vi "ReadMicaCSV.vi"() -> ()   [LabVIEW 2018]
uses:
  <vilib>/ErrorRing/Error Ring.xnode
panel:
  in  "選資料":u16(ring) items=["M27MRH01        ", "VM-POR-01TSU1   ", "VM-POR-BRGTWS   ", "VM-TRE-BRGTWS   ", "VM-TRE-BRGTDS   ", "VM-MDR-01BRGTWS ", "VM-MDR-01BRGTDS ", "VM-MDR-01TSI1   ", "VM-POR-01PLG    ", "LTRVLTFBT1      ", "LTRCURFBT1      ", "LTRSPFBT1       ", "VM-MDR-01IMFB2  ", "MILVLTFBT1      ", "MILCURFBT1      ", "MILSPFBT1       ", "RTRCURFBT1      ", "RTRSPFBT1       ", "VM-POR-01VTFB   ", "VM-POR-01IMFB   ", "W14ILTR         ", "W22ILTR         ", "W41OTDRV        ", "LSMSPFBT1       ", "RSMSPFBT1       ", "WB3AI0T1        ", "W21OTDRV        ", "WSRFT1          ", "DSRFT1          ", "W02DIATN        ", "W03DIATN        ", "W00LTRD1        ", "M30MRH01        ", "M31MRH01        ", "M32MRH01        ", "M33MRH01        ", "M34MRH01        ", "M36MRH01        ", "M40MRH01        ", "MRHRIL          ", "M17MRH01        ", "M04RTDIA        ", "M04LTDIA        ", "MMILBYTE        ", "W06MRH          ", "D10RTDIA!       ", "M00ASD03        ", "M01ASD03        ", "M02ASD03        ", "M04ASD03        ", "M05ASD03        ", "M01TSLTR        ", "T01TSLTR        ", "M00TSLTR        ", "M32STBR1        ", "M80TSLTR        ", "M07TAILTRK      ", "M08MRH01        ", "STBRMEM         ", "SPLITMEM        ", "M91RCON1        ", "M09RCON1        ", "M19RCON1        ", "M15RCON1        ", "M21RCON1        ", "M17RCON1        ", "M13RCON1        ", "M61RCON2        ", "M50RCON2        ", "MMILSPIN        ", "M20LTDIA        ", "W22IRTR         ", "W10TCOMP        ", "W17IRTR         ", "W17ILTR         ", "W02AI0T1        ", "W06AI0T1        ", "W11RTDIA        ", "M71HEADTRK      ", "M01SVC01        ", "M05SVC01        ", "M03SSPT         ", "PX-MDR-03       ", "MTHRREF         ", "MSQTHR01        ", "MMDGAPOPN       ", "MMDGAPCLS       ", "MPORTSTAR       ", "PSRSPFB1        ", "M02SVC01        ", "M13LTDIA        ", "M04TAILTRK      ", "M81TAILTRK      ", "MSTRATESLTR     ", "MMSTATESRTR     ", "WSREFATESRTR    ", "MATESRTRSTOP    ", "KSTP-LINE       ", "M24STBR1        ", "M17STBR1        ", "M18STBR1        ", "MA6STBR1        ", "M19STBR1        ", "W16IRTR         ", "QSTP-MILLMSW    ", "NSTP-MILLMSW    ", "M01MRH01        ", "M05MRH01        ", "M32ASD04        ", "W10ASD03        ", "DA4ASD03!       ", "MSTRATESRTR     ", "MTRWINDRF       ", "MPORWINDRF      ", "MTROGAPRF       ", "DXR-MATE-ON     ", "M04ATESRTR      ", "M12TAILTRK      ", "M13TAILTRK      ", "M01SSPT         ", "W24IRTR         ", "W00TSRTR        ", "CPCACTSDEV      ", "CPCACTCYL       ", "W32TCOMP        ", "W33TCOMP        ", "W25TCOMP        ", "W26TCOMP        ", "M21THR01        ", "M40THR01        ", "M43THR01        ", "M50THR01        ", "M03TOUT1        ", "M11RCON1        ", "M35RCON1        ", "M27RCON1        ", "M01JGMIL        ", "M08JGMIL        ", "M11JGMIL        ", "WPC30C2E        ", "M18JGMIL        ", "WRBEND          ", "IMRBEND         ", "W36AUXACR2      ", "W24AUXACR2      ", "EXR-TRV-MSR     ", "EXR-TRV-SRV     ", "EXR-TRV-CHECK   ", "EXR-OPN         ", "DXR-TRV-MSR     ", "DXR-TRV-SRV     ", "DXR-TRV-CHECK   ", "DXR-OPN         ", "SSA-MEG-01AR    ", "SSA-MEG-03AR    ", "SSA-MEG-09AR    ", "SSA-MEG-12AR    ", "WL2SCHTHICK     ", "NML-MILDBR1     ", "NML-MILDBR2     ", "W17AI0T1        ", "W16AI0T1        ", "W01ZRHY         ", "WIIH1CPCDEV     ", "WRWSBEND        ", "WRDSBEND        ", "ESPDSP          ", "DSPDSP          ", "WPORDIA         ", "W61ILTR         ", "W02PDATA        ", "MX1ECMP         ", "MX1DCMP         ", "W11TCOMP        ", "M04TCOMP        ", "M05TCOMP        ", "DXR-CLS         ", "M17RTDIA        ", "DXR-MSR-RQ      ", "EXR-MSR-RQ      ", "PX-MDG-21       ", "D3H-MDG-04AR    ", "VM-TRE-01IMFB   ", "RTRIMFBT2       ", "MILIMFBT2       ", "RTRVLTFBT2      ", "W50ACTDT        ", "M00TSRTR        ", "QSTOP           ", "W12HEADTRK      ", "WA1HEADTRK      ", "WB1HEADTRK      ", "W12TAILTRK      ", "W22TAILTRK      ", "M80DIATN        ", "M40ASD04        ", "M25MRH01        ", "MASDCTLD1       ", "M01ASDCK        ", "M03ASDCK        ", "M04ASDCK        ", "W06TCOMP        ", "W29AUXACR2      ", "RSMCURFBT1      ", "LSMCURFBT1      ", "W04TCOMP        ", "W31ATRVREF      ", "M12ATRVREF      ", "MPORASRMD       ", "MREWASRMD       ", "W31ASRTREF      ", "W22ATRVREF      ", "M06TSRTR        ", "W22ASRTREF      ", "W21ASRTREF      ", "VM-TRE-0152AB   ", "VM-TRE-01HF     ", "VM-TRE-01RON    ", "VM-POR-0152AB   ", "VM-POR-01HF     ", "VM-POR-01RON    ", "VM-MDR-0152AB   ", "VM-MDR-01HF     ", "VM-MDR-01RON    ", "M39RCON2        ", "W11OTDRV        ", "W31OTDRV        ", "W51OTDRV        ", "M22BRKDT        ", "M01IBRTR        ", "M14JGTAN1       ", "M14JGTAN3       ", "M04JGLTR        ", "M07JGLTR        ", "M06JGLTR        ", "M01JGLTR        ", "WN12827|4       ", "MPLNML          ", "MPLWEDGRET      ", "ROLMODERW       ", "M46RCON1        ", "PX-POR-04       ", "M08ROLGAP       ", "ROLMODENLR      ", "M70RCON1        ", "WN12826|10      ", "MMILLGRLO       ", "MMILLGRHI       ", "FS-MDR-01       ", "M16JGMIL        ", "M17JGMIL        ", "WPC20B01|1      ", "M47RCON1        ", "D2H-6UM-01AR    ", "D2H-6UM-02AR    ", "W02AI0T11       ", "W04AI0T11       ", "W06AI0T11       ", "W08AI0T11       ", "W53SSPT         ", "VM-MDR-0170AB   ", "W08PORSPC       ", "W11PORSPC       ", "W07PORSPC       ", "M03PORSPC       ", "FWDDRAFT        ", "BWDDRAFT        ", "M16MRH01        ", "PS-PUH-01TD     ", "PX-MEG-10       ", "VM-POR-01NRF    ", "N12AE6          ", "GERDTLTR        ", "W33DWDTP        ", "W76AUXACR2      ", "DELTMFB-DEV     ", "ENTTMFB-DEV     ", "W80DIATN        ", "D30ASD02!       ", "M14ASD03        ", "W80IDATA        ", "DASDREMLEN!     ", "M12RTDIA        ", "W24DIATN        ", "D45CNTB1!       ", "W14LTDIA        ", "DA1ACTDT!       ", "WF2ACTDT        ", "M31ASD04        ", "M02ASD04        ", "M34ASD04        ", "M01ASD04        ", "D3A-MDG-05AR    ", "D3A-MDG-05BR    ", "WLHTENFBT3      ", "WRHTENFBT3      ", "W0BAI0T31       ", "W0CAI0T31       ", "D32ASD02!       ", "D33ASD02!       ", "MMDGAPC         ", "W03PORANGL      ", "CPC-AUTO1       ", "M03SVC01        ", "W09AI0T31       ", "W92TCOMPT3      ", "W93TCOMPT3      ", "D11LTRD3!       ", "MA1BRKDT        ", "WN12809|9       ", "CPCLARGEALM     ", "PS-POR-01       ", "PS-TRE-01TD     ", "WDL146L|4       ", "M48ASD04        ", "M06ASD03        ", "W60L2M03A       ", "W61L2M03A       ", "W41IDATA        ", "W09ASDCK        ", "W08ASDCK        ", "M08ASDCK        ", "M42DIATN        ", "M10LTRD3        ", "W01LTRD3        ", "W06ADCK         ", "M06RTDIA        ", "M10RTDIA        ", "M23RTDIA        ", "M06ASDCK        ", "W10ASDCK        ", "D04ASD03!       ", "D05ASD02!       ", "W04AUXACR2      ", "MA4STBR1        ", "MA5STBR1        ", "MA0STBR1        ", "MA1STBR1        ", "M23CDATA        ", "W47CDATA        ", "M13ASDCK        ", "M11ASDCK        ", "W13ASDCK        ", "M17ASDCK        ", "WLDPOROD        ", "D05ASD03!       ", "M21MRH01        ", "D2H-6UM-09AR    ", "MAUDLIFT        ", "D3H-6UM-01AR    ", "T04ATESRTR      ", "W12ATESRTR      ", "W15ATESRTR      ", "M02TAILTRK      ", "W16ATESRTR      ", "M93TAILTRK      ", "W23TAILTRK      ", "W13TAILTRK      ", "M09ATESRTR      ", "M32RCON1        ", "M52M-TRE        ", "M52M-MDR        ", "M52M-POR        ", "M19ASD03        ", "W21ASDCK        ", "W17ASDCK        ", "F01ASD03%       ", "D12LTRD3!       ", "DELTMFBT3       ", "W30LTRD3        ", "D30LTRD3!       ", "M05LTRD3        ", "D09ASD03!       ", "M20LTRD3        ", "D53LTRD3!       ", "M33LTRD3        ", "VM-MDR-01NRF    ", "MSTR-BRAKE      ", "FE-STR-MB       ", "FE-STR-MILL     ", "W35AUXACR2      ", "W01DWDT         ", "W03DWDT         ", "M51IRTR         ", "M02STBR1        ", "WN1281D|1       ", "W51AUXACR1      ", "W25HEADTRK      ", "M62HEADTRK      ", "VM-MDG-01IRF    ", "M52MRH01        ", "VM-MDG-01NRF    ", "W31AUXACR2      ", "M37RCON1        ", "W16ILTR         ", "W66TCOMP        ", "W70TCOMP        ", "W21AIOT1        ", "M00AIOT1        ", "LTRROTFBT1      ", "W20AIOT1        ", "VM-POR-01NFB    ", "W52TCOMP        ", "M50TCOMP        ", "W11LTDIA        ", "W24TENFB        ", "W14TENFB        ", "WA1ATRVREF      ", "W20IRTR         ", "W14IRTR         ", "M86DIATN        ", "W32IRTR         ", "WBWLOSS         ", "W20ILTR         ", "W70DIATN        ", "PX-BWR-01       ", "PX-BWR-02       ", "RTRROTFBT1      ", "W25IRTR         ", "M02LTRD1        ", "M47DIATN        ", "RTRMDROTFBT1    ", "F23DWDT%        ", "WK3IRTR         ", "M50MECHREW      ", "W92MECHREW      ", "WN129C4|6       ", "M06BWLOS        ", "M12LTRD3        ", "W31TCOMP        ", "M20TCOMP        ", "M22TCOMP        ", "W42TAPERTRK     ", "M31TAPERTRK     ", "W63MRH          ", "LSLDRAFT        ", "W15AGCVREF      ", "VM-MDG-01NFB    ", "VM-MDG-01IFB    ", "W11ZRHY         ", "VM-TRE-01NRF    ", "W01BWLOS        ", "PWC-IW-LOWER    ", "SSA-CLS-01AR    ", "F04IRTR%        ", "W11MRH          ", "M21ACRCHG       ", "M02ACRCHG       ", "M03TSRTR        ", "RSLDRAFT        ", "W54AUXACR2      ", "W53AUXACR2      ", "D3H-TRE-01AR    ", "W95ACTDT        ", "W96ACTDT        ", "EXR-FLT         ", "DXR-FLT         ", "M02HF01         ", "W55OTDRV        ", "W52OTDRV        ", "W09PORSPC       ", "W56OTDRV        ", "W23ATESLTR      ", "MILL-ETJABX1    ", "MG4JGTAN4       ", "VM-TRE-01NFB    ", "VM-TRE-01IFB    ", "VM-TRE-01PLG    ", "W90MECHREW      ", "W91MECHREW      ", "M36TAILTRK      ", "M41ASD03        ", "M25ASD04        ", "M40ASD03        ", ""]
  in  "選檔案":u16(ring) items=["...", "lot1_s1_iron0_p1.csv", "lot1_s2_iron0_p1_shift.csv", "lot2_s1_iron1_p1.csv", "lot2_s2_iron1_p1.csv", "lot3_s1_iron1_p2.csv", "lot3_s2_iron1_p3.csv", "ton_0_p0_2.csv", "ton_10_p0.csv", "ton_8_p0.csv"]
  in  "Load":bool
  in  "資料夾":path=path "G:/共用雲端硬碟/All-mechatronics/中鋼專區/中鋁壓延量測/Mica_Rawcsv"
  out "Waveform Graph":dbl[](graph)
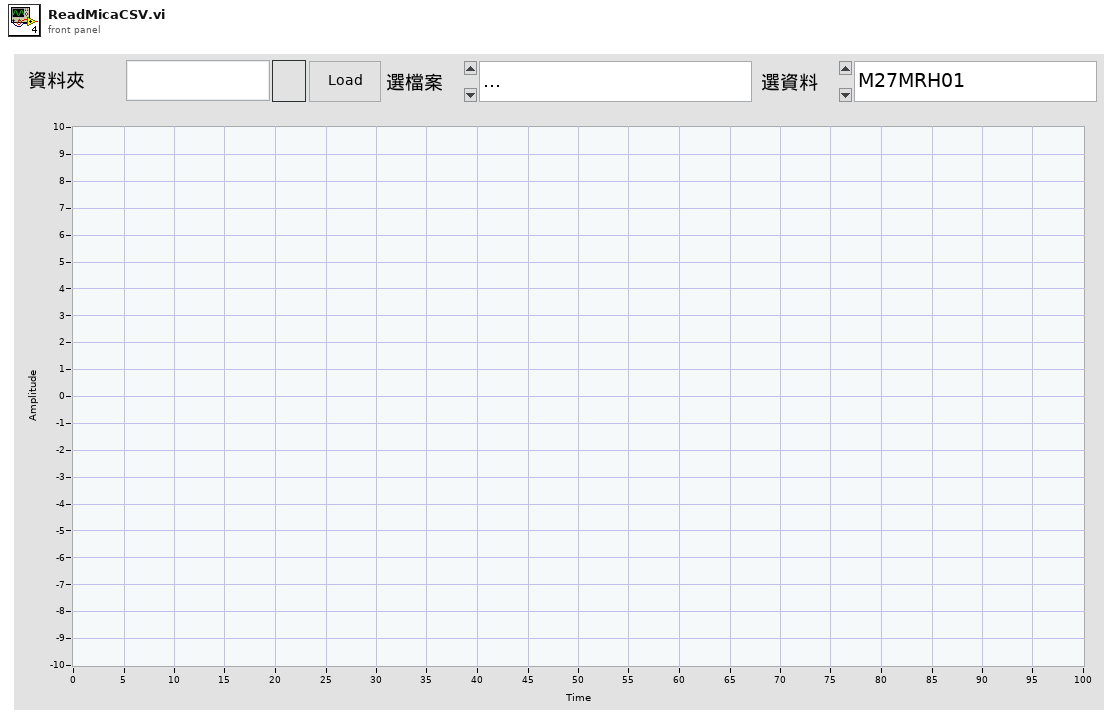
[diagram p1: front panel]
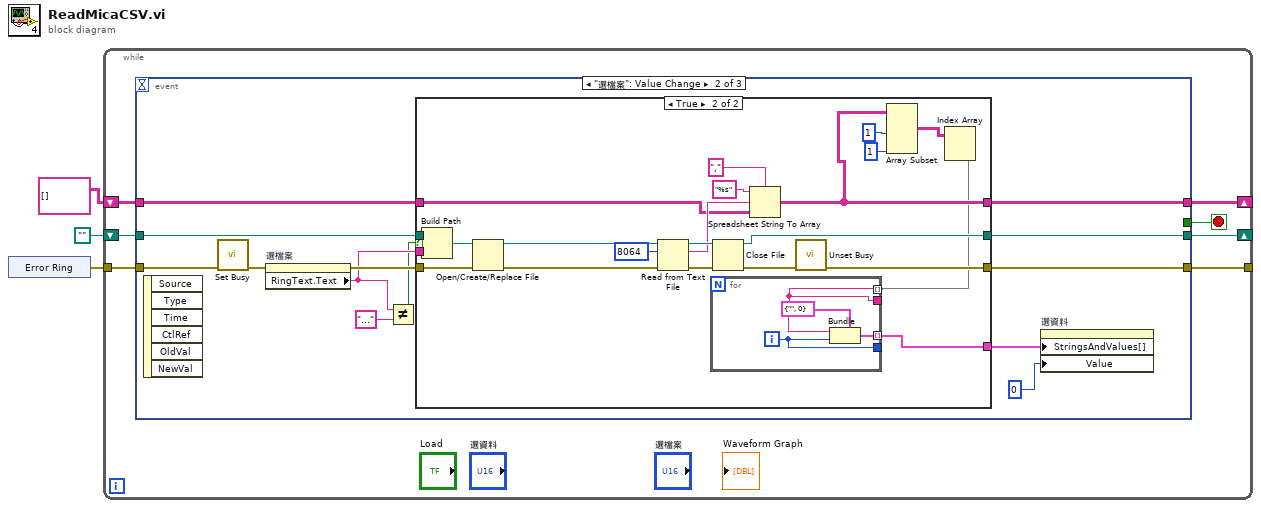
[diagram p0: block diagram]
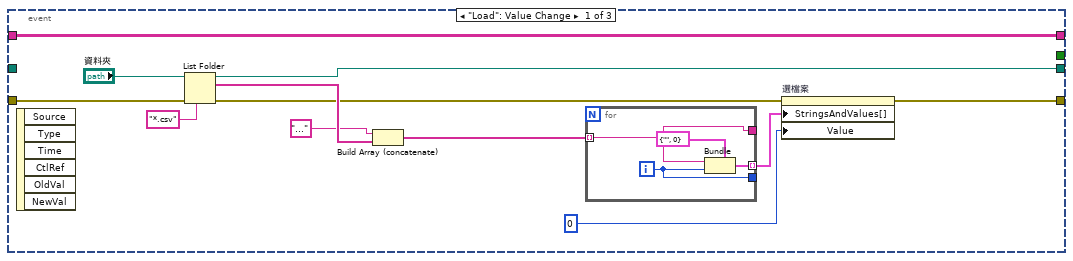
[diagram p2: hidden frame]
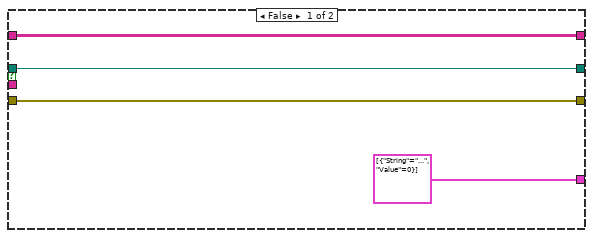
[diagram p3: hidden frame]
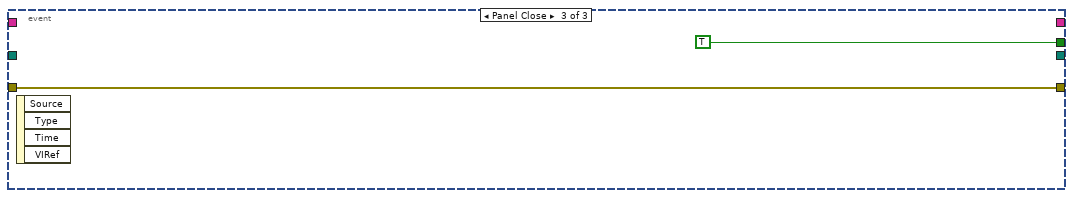
[diagram p4: hidden frame]
diagram:
  n1 = xnode "Error Ring"() -> ("error out"=w3:errorcluster)
  n2 = while {
    tunnel: w3 -> [w9]
    tunnel: [w8] -> _
    shift-right: [w6] -> _
    shift-left: path "" -> [w7]
    shift-right: [w4] -> _
    shift-left: string[][] [] -> [w5]
    stop <- w10 stop-if-true
    n3 = event shown="[1] \"選檔案\": Value Change" {
      selector: _ -> [_ _ _]
      dyn-events: _ -> [_ _ _]
      timeout: _ -> [_ _ _]
      tunnel: [_ _ TRUE] -> w10
      tunnel: w9 -> [w15 w39 w70]
      tunnel: [w13 w37 w70] -> w8
      tunnel: w7 -> [_ w35 _]
      tunnel: [w11 w38 _] -> w6
      tunnel: w5 -> [w12 w36 _]
      tunnel: [w12 w32 _] -> w4
      event "Load": Value Change {
        n4 = event-data() -> ()  [unwired: 1 in, 6 out]
        n5 = List Folder(path="資料夾", pattern="*.csv", error in=w15) -> (path out=w11:path, filenames=w21:string[], error out=w14:errorcluster)  [unwired: 1 in, 1 out]
        n6 = Build Array (concatenate)("..." ("element"), w21) -> (w20:string[])
        n7 = for {
          tunnel: [w26] -> w18 mode=indexing
          tunnel: w20 -> [w23] mode=indexing
          tunnel: [w24] -> _
          tunnel: [w23] -> _
          i -> [w24]
          n8 = Bundle(cluster=cluster{"String":string, "Value":u16} {"String"="", "Value"=0}, "String"=w23, "Value"=w24) -> (w26:cluster{"String":string, "Value":u16})
        }
        n9 = property on="選檔案" class="Ring (strict)"(error in=w14, "StringsAndValues[]"=w18, "Value"=u16 0) -> (error out=w13:errorcluster)  [unwired: 1 in, 1 out]
      }
      event "選檔案": Value Change {
        n10 = event-data() -> ()  [unwired: 1 in, 6 out]
        n11 = call <vilib>:"Set Busy.vi"("error in (no error)"=w39) -> ("error out"=w34:errorcluster)  [unwired: 9 in, 1 out]
        n12 = property on="選檔案" class="Ring (strict)"(error in=w34) -> (error out=w33:errorcluster, "RingText.Text"=w30:string)  [unwired: 1 in, 1 out]
        n13 = Not Equal?(x=w30, y="...") -> (x != y?=w27:bool)
        n14 = case shown="True" w27 {
          tunnel: [w41 w61] -> w38
          tunnel: [w42 w60] -> w37
          tunnel: w36 -> [w40 w57]
          tunnel: w35 -> [w41 w55]
          tunnel: w33 -> [w42 w54]
          tunnel: [w40 w50] -> w32
          tunnel: [cluster{"String":string, "Value":u16}[] [{"String"="...", "Value"=0}] w48] -> w31
          tunnel: w30 -> [_ w47]
          frame False {
          }
          frame True {
            n15 = Build Path(base path=w55, name or relative path=w47) -> (appended path=w53:path)
            n16 = Open/Create/Replace File(file path (use dialog)=w53, error in=w54) -> (refnum out=w45:refnum<file>, error out=w65:errorcluster)  [unwired: 4 in, 1 out]
            n17 = Read from Text File(file (use dialog)=w45, count=8064, error in=w65) -> (refnum out=w64:refnum<file>, text=w59:string, error out=w63:errorcluster)  [unwired: 1 in, 1 out]
            n18 = Close File(refnum=w64, error in=w63) -> (path=w61:path, error out=w62:errorcluster)
            n19 = Spreadsheet String To Array(delimiter (Tab)=",", format string="%s", spreadsheet string=w59, array type (2D Dbl)=w57) -> (array=w50:string[][])
            n20 = call <vilib>:"Unset Busy.vi"("error in (no error)"=w62) -> ("error out"=w60:errorcluster)  [unwired: 10 in]
            n21 = Array Subset(array=w50, length (row)=1 ("length"), index (col)=1 ("index")) -> (w51:string[][])  [unwired: 2 in]
            n22 = Index Array(array=w51) -> (element=w49:string[])  [unwired: 2 in]
            n23 = for {
              tunnel: [w69] -> w48 mode=indexing
              tunnel: [w67] -> _
              tunnel: [w66] -> _
              tunnel: w49 -> [w66] mode=indexing
              i -> [w67]
              n24 = Bundle(cluster=cluster{"String":string, "Value":u16} {"String"="", "Value"=0}, "String"=w66, "Value"=w67) -> (w69:cluster{"String":string, "Value":u16})
            }
          }
        }
        n25 = property on="選資料" class="Ring (strict)"("StringsAndValues[]"=w31, "Value"=u16 0) -> ()  [unwired: 2 in, 2 out]
      }
      event Panel Close {
        n26 = event-data() -> ()  [unwired: 1 in, 4 out]
      }
    }
  }
